vi "UHR-Fleezers Control (host) - 12.0_test_fpga_connection.vi"() -> ()   [LabVIEW 2014] (continued)
              n285 = Add(x=w488, y="Osc. center (V)") -> (x+y=w486:dbl)
              n286 = Divide(x=w486, y=10.0) -> (x/y=w484:dbl)
              n287 = Multiply(x=w484, y=32767.0) -> (x*y=w479:dbl)
              n288 = Select(t=w479, s="Scan axis", f=w499) -> (s? t:f=w497:dbl)
              n289 = Select(t=w498, s="Scan axis", f=w479) -> (s? t:f=w496:dbl)
              n290 = local read "MCL Mode"() -> (w478:u16)
              n291 = Not Equal?(x=w478, y=u16 1) -> (x != y?=w475:bool)
              n292 = local read "Stop All"() -> (w476:bool)
              n293 = xnode "Read/Write Control"("FPGA VI Reference In"=w512, "AO1"=w497, "AO2"=w496) -> ()  [unwired: 1 in, 2 out]
              n294 = Compound Arithmetic op=OR(w476, w475) -> (w474:bool)
              n295 = node-c288() -> ()  [unwired: 2 out]
            }
            n296 = node-c288(w472) -> ()  [unwired: 1 out]
          }
          frame 2 {
            n297 = case shown="True" "Start Scan" {
              tunnel: w518 -> [_ w530]
              frame False {
              }
              frame True {
                n298 = Subtract(x="End (V)", y="Begin (V)") -> (x-y=w526:dbl)
                n299 = Decrement(x="N Points") -> (x-1=w525:dbl)
                n300 = Divide(x=w526, y=w525) -> (x/y=w523:dbl)
                n301 = for {
                  N: "N Points" -> [_]
                  tunnel: "Begin (V)" -> [w543]
                  tunnel: w530 -> [w535]
                  tunnel: [w534] -> w529 mode=indexing
                  tunnel: w523 -> [w533]
                  tunnel: [w531] -> w522 mode=indexing
                  i -> [w542]
                  n302 = Multiply(x=w533, y=w542) -> (x*y=w541:dbl)
                  n303 = Add(x=w543, y=w541) -> (x+y=w538:dbl)
                  n304 = local read "Scan axis"() -> (w532:bool)
                  n305 = local read "AO1"() -> (w540:dbl)
                  n306 = local read "AO2"() -> (w539:dbl)
                  n307 = Select(t=w538, s=w532, f=w540) -> (s? t:f=w537:dbl)
                  n308 = Select(t=w539, s=w532, f=w538) -> (s? t:f=w536:dbl)
                  n309 = flat-sequence {
                    tunnel: w537 -> [w547]
                    tunnel: w536 -> [w546]
                    tunnel: w535 -> [w544]
                    tunnel: [w557] -> w534
                    tunnel: [w556] -> w531
                    frame #0 {
                      w550 = 10.0 ("y")
                      w545 = 32767.0 ("y")
                      n310 = Multiply(x=w547, y=w545) -> (x*y=w553:dbl)
                      n311 = Multiply(x=w546, y=w545) -> (x*y=w551:dbl)
                      n312 = Divide(x=w553, y=w550) -> (x/y=w554:dbl)
                      n313 = Divide(x=w551, y=w550) -> (x/y=w552:dbl)
                      n314 = To Word Integer(number=w554) -> (16bit integer=w548:i16)
                      n315 = To Word Integer(number=w552) -> (16bit integer=w549:i16)
                      n316 = xnode "Read/Write Control"("FPGA VI Reference In"=w544, "AO1"=w548, "AO2"=w549) -> ()  [unwired: 1 in, 2 out]
                    }
                    frame #1 {
                      n317 = Wait (ms)(milliseconds to wait="DAQ Delay (ms)") -> ()  [unwired: 1 out]
                    }
                    frame #2 {
                      n318 = local read "Slow mean"() -> (w557:dbl)
                      n319 = local read "Sigma"() -> (w556:dbl)
                    }
                  }
                }
                n320 = Bundle("Begin (V)"="Begin (V)", w523, w529) -> (→"MCL Scan":cluster{"Begin (V)":dbl, dbl, dbl[]})  [unwired: 1 out]
                n321 = Bundle("Begin (V)"="Begin (V)", w523, w522) -> (→"MCL Scan 2":cluster{"Begin (V)":dbl, dbl, dbl[]})  [unwired: 1 out]
              }
            }
          }
        }
        n322 = local read "Stop All"() -> (w467:bool)
        n323 = node-c288() -> ()  [unwired: 2 out]
      }
      n324 = node-c288(w464) -> ()  [unwired: 1 out]
    }
    frame Enabled {
    }
  }
  n325 = node-c288(3 ("Processor")) -> (w135:T26)  [unwired: 3 out]
  n326 = timed-loop "Oscillate Trap/AOM (fishing, debugging)" {
    tunnel: w51 -> [w561]
    tunnel: [w560] -> w140
    timing: w135 -> [_]
    timing-out: [_] -> w134
    stop <- w560 stop-if-true
    n327 = node-c288() -> ()  [unwired: 2 out]
    n328 = event shown="[0] \"Oscillate Set 1\", \"Fish\": Value Change" {
      selector: _ -> [_ _ _]
      dyn-events: _ -> [_ _ _]
      timeout: _ -> [_ _ _]
      tunnel: w561 -> [w568 _ _]
      tunnel: [FALSE ("Stop All") _ w1253] -> w560
      event "Oscillate Set 1", "Fish": Value Change {
        n329 = event-data() -> ()  [unwired: 6 out]
        n330 = local read "Oscillate Set 1"() -> (w567:bool)
        n331 = Or(x=w567, y="Fish") -> (x .or. y?=w565:bool)
        n332 = case shown="True" w565 {
          tunnel: w568 -> [_ w571]
          tunnel: "Fish" -> [_ w569]
          frame False {
          }
          frame True {
            n333 = case shown="True" w569 {
              selector: w569 -> [w574 w575]
              tunnel: [w574 w575] -> w570
              frame False {
              }
              frame True {
                w576 = FALSE ("Tether")
                n334 = local write "Scan axis 2"(TRUE) -> ()
                n335 = local write "Tether"(w576) -> ()
                n336 = local write "Hysteresis"(w576) -> ()
                n337 = local write "Multiple tether"(w576) -> ()
                n338 = local write "Bad fit"(w576) -> ()
                n339 = local write "Good tether"(w576) -> ()
                n340 = property on="Trap D (MHz)" class="DigNum (strict)"("Val(Sgnl)"="Furthest D (MHz)") -> ()  [unwired: 2 in, 2 out]
                n341 = local read "Flow ON\nduring cal?"() -> (w577:bool)
                n342 = Or(x="Flow ON during \nfishing?", y=w577) -> (x .or. y?=w578:bool)
                n343 = Wait (ms)(milliseconds to wait=u32 500) -> ()  [unwired: 1 out]
                n344 = property on="Sample Channel\nFlow" class="Bool (strict)"("Val(Sgnl)"=w578) -> ()  [unwired: 2 in, 2 out]
              }
            }
            n345 = node-c288() -> (w573:T26)  [unwired: 4 out]
            n346 = timed-loop "Oscillate AOD" {
              timing: w573 -> [_]
              timing-out: [_] -> w572
              tunnel: w571 -> [w590]
              tunnel: w570 -> [w584]
              i -> [w592]
              stop <- w583 stop-if-true
              n347 = node-c288() -> (w591:i64)  [unwired: 1 out]
              n348 = flat-sequence {
                tunnel: w592 -> [w619]
                tunnel: w591 -> [w618]
                tunnel: w590 -> [w597]
                tunnel: w584 -> [w600]
                tunnel: [w600] -> w589
                tunnel: [w599] -> w588
                tunnel: [w596] -> w587
                tunnel: [w593] -> w585
                tunnel: w589 -> [w662]
                tunnel: w588 -> [w660]
                tunnel: w587 -> [w659]
                tunnel: [w658] -> w586
                tunnel: w585 -> [w657]
                tunnel: [w818] -> w583
                tunnel: w586 -> [w817]
                frame #0 {
                  n349 = Divide(x=w618, y=i64 1000) -> (x/y=w613:dbl)
                  n350 = Multiply(x=w613, y=w619) -> (x*y=w615:dbl)
                  n351 = local read "BD 1 Frequency 2 (MHz)"() -> (w598:dbl)
                  n352 = Multiply(x="Osc. freq. (Hz)", y=6.283185307179586) -> (x*y=w616:dbl)
                  n353 = Multiply(x=w616, y=w615) -> (x*y=w595:dbl)
                  n354 = local read "BD 1 Frequency 1 (MHz)"() -> (w603:dbl)
                  n355 = local read "BD 2 Frequency 1 (MHz)"() -> (w602:dbl)
                  n356 = case shown="True" w600 {
                    tunnel: w595 -> [w625 w630]
                    tunnel: w603 -> [_ w641]
                    tunnel: w598 -> [_ w642]
                    tunnel: [w622 w636] -> w601
                    tunnel: [FALSE w633] -> w596
                    tunnel: [0.0 w626] -> w593
                    frame False {
                      n357 = Sine(x=w625) -> (sin(x)=w623:dbl)
                      n358 = Multiply(x=w623, y="Osc. amp. (MHz)") -> (x*y=w622:dbl)
                    }
                    frame True {
                      n359 = Cosine(x=w630) -> (cos(x)=w645:dbl)
                      n360 = Subtract(x=w642, y=w641) -> (x-y=w640:dbl)
                      n361 = Decrement(x=w645) -> (x-1=w644:dbl)
                      n362 = Subtract(x=w640, y="Closest D (MHz)") -> (x-y=w637:dbl)
                      n363 = Divide(x=w644, y=-2.0) -> (x/y=w638:dbl)
                      n364 = Multiply(x=w638, y=w637) -> (x*y=w636:dbl)
                      n365 = local read "Vec Mean of T1 T2"() -> (w632:dbl[])
                      n366 = Greater?(x=w632, y="Stop F (pN)") -> (0:w634:bool[])
                      n367 = Or Array Elements(Boolean array=w634) -> (logical OR=w633:bool)
                      n368 = Divide(x=w630, y=6.283185307179586) -> (x/y=w629:dbl)
                      n369 = Round Toward +Infinity(x=w629) -> (ceil(x): smallest int >= x=w626:dbl)
                      "Attempts" <- w626
                      n370 = Greater?(x=w626, y="Attempt Limit") -> (0:w628:bool)
                      n371 = case shown="True" w628 {
                        frame False {
                        }
                        frame True {
                          n372 = local write "Fish"(FALSE ("Fish for Tether")) -> ()
                          n373 = local read "Messages"() -> (w647:string)
                          n374 = flat-sequence {
                            frame #0 {
                              n375 = call <vilib>:"Beep.vi"("use system alert? (T)"=FALSE, "duration (msec)"=u32 200, "frequency (Hz)"=u32 500) -> ()  [unwired: 9 out]
                            }
                            frame #1 {
                              n376 = Wait (ms)(milliseconds to wait=u32 100) -> ()  [unwired: 1 out]
                            }
                            frame #2 {
                              n377 = call <vilib>:"Beep.vi"("use system alert? (T)"=FALSE, "duration (msec)"=u32 200, "frequency (Hz)"=u32 500) -> ()  [unwired: 9 in]
                            }
                          }
                          n378 = call "Update messages.vi"("Message to add"="Tether fishing timeout." ("Messages"), "Old message string"=w647) -> ("New message string"=→"Messages":string)
                        }
                      }
                    }
                  }
                  n379 = Select(t=w603, s="Scan axis 2", f=w602) -> (s? t:f=w606:dbl)
                  n380 = Add(x=w601, y=w606) -> (x+y=w599:dbl)
                  n381 = Select(t=w599, s="Scan axis 2", f=w603) -> (s? t:f=w609:dbl)
                  n382 = Select(t=w602, s="Scan axis 2", f=w599) -> (s? t:f=w608:dbl)
                  n383 = local read "Y RF Frequency Limits (MHz)"() -> (w604:T17)
                  n384 = local read "X RF Frequency Limits (MHz)"() -> (w605:T17)
                  n385 = local read "BD 2 Frequency 2 (MHz)"() -> (w611:dbl)
                  n386 = local read "BD 2 Frequency 3 (MHz)"() -> (w610:dbl)
                  n387 = local read "BD 1 Frequency 3 (MHz)"() -> (w612:dbl)
                  n388 = call "set RF board frequency - interlace.vi"("Board 2 Frequency Limits"=w604, "Board 1 Frequency Limits"=w605, "FPGA VI Reference In"=w597, "Board 2 Frequency 3 (MHz)"=w610, "Board 1 Frequency 3 (MHz)"=w612, "Board 2 Frequency 2 (MHz)"=w611, "Board 2 Frequency 1 (MHz)"=w608, "Board 1 Frequency 2 (MHz)"=w598, "Board 1 Frequency 1  (MHz)"=w609) -> ()  [unwired: 1 in, 2 out]
                }
                frame #1 {
                  n389 = And(x=w662, y=w659) -> (x .and. y?=w661:bool)
                  n390 = case "Only if were fishing and now formed tether" shown="True" w661 {
                    tunnel: w660 -> [w664 w679]
                    tunnel: [w663 w678] -> w658
                    tunnel: w657 -> [_ w674]
                    frame False {
                      n391 = local read "Fish"() -> (w663:bool)
                      n392 = case shown="False" w663 {
                        tunnel: w664 -> [w665 _]
                        frame False {
                          n393 = property on="BD 1 Frequency 1 (MHz)" class="DigNum (strict)"("Val(Sgnl)"=w665) -> ()  [unwired: 2 in, 2 out]
                        }
                        frame True {
                        }
                      }
                    }
                    frame True {
                      w678 = FALSE ("Fish for Tether")
                      n394 = call <vilib>:"Beep.vi"() -> ()  [unwired: 3 in, 9 out]
                      n395 = Number To Decimal String(number=w674, width (-)=i16 1) -> (decimal integer string=w672:string)
                      n396 = Concatenate Strings("Formed tether in ", w672, " attempt(s)." ("string")) -> (w669:string)
                      n397 = local read "Messages"() -> (w676:string)
                      n398 = local write "Fish"(w678) -> ()
                      n399 = call "Update messages.vi"("Message to add"=w669, "Old message string"=w676) -> ("New message string"=w675:string)
                      n400 = local write "Messages"(w675) -> ()
                      n401 = Get Date/Time In Seconds() -> (seconds since 1Jan1904=→"Time tether formed":timestamp)
                      n402 = local read "Flow ON\nduring cal?"() -> (w666:bool)
                      n403 = property on="Sample Channel\nFlow" class="Bool (strict)"("Val(Sgnl)"=w666) -> (error out=w667:errorcluster)  [unwired: 2 in, 1 out]
                      n404 = case shown="\"2\", \"3\", \"4\", \"5\", \"6\"" "Then..." {
                        selector: "Then..." -> [_ w682 _ _]
                        tunnel: w679 -> [w681 _ _ _]
                        tunnel: w667 -> [_ _ _ _]
                        frame "1", Default {
                          n405 = property on="BD 1 Frequency 1 (MHz)" class="DigNum (strict)"("Val(Sgnl)"=w681) -> ()  [unwired: 2 in, 2 out]
                        }
                        frame "2", "3", "4", "5", "6" {
                          n406 = flat-sequence {
                            tunnel: w682 -> [w688]
                            frame #0 {
                              n407 = local read "Flow ON\nduring cal?"() -> (w683:bool)
                              n408 = property on="Sample Channel\nFlow" class="Bool (strict)"("Val(Sgnl)"=w683) -> ()  [unwired: 2 in, 2 out]
                              n409 = property on="Trap D (MHz)" class="DigNum (strict)"("Val(Sgnl)"="Move to D 1 (MHz)") -> ()  [unwired: 2 in, 2 out]
                            }
                            frame #1 {
                              n410 = local read "Wait Before Save (s)"() -> (w685:u32)
                              n411 = Multiply(x=u32 1000 ("milliseconds to wait"), y=w685) -> (x*y=w687:u32)
                              n412 = Wait (ms)(milliseconds to wait=w687) -> ()  [unwired: 1 out]
                            }
                            frame #2 {
                              n413 = case shown="\"5\", \"6\"" w688 {
                                selector: w688 -> [w691 w701 _]
                                frame "3", "4" {
                                n414 = flat-sequence {
                                tunnel: w691 -> [w692]
                                tunnel: [w692] -> w689
                                tunnel: [w694] -> w690
                                tunnel: w689 -> [w694]
                                tunnel: w690 -> [w698]
                                frame #0 {
                                n415 = property on="Green ON/Interlacing" class="Bool (strict)"("Val(Sgnl)"=TRUE ("Value (Signaling)")) -> ()  [unwired: 2 in, 2 out]
                                }
                                frame #1 {
                                n416 = Multiply(x="Wait Before Save (s)", y=u32 1000 ("x")) -> (x*y=w696:u32)
                                n417 = Wait (ms)(milliseconds to wait=w696) -> ()  [unwired: 1 out]
                                }
                                frame #2 {
                                n418 = property on="Start Saving" class="Bool (strict)"("Value"=TRUE ("Start Saving")) -> ()  [unwired: 2 in, 2 out]
                                n419 = case shown="\"4\"" w698 {
                                frame Default {
                                }
                                frame "4" {
                                n420 = property on="Fl. Triggered..." class="Bool (strict)"("Val(Sgnl)"=TRUE ("Value (Signaling)")) -> ()  [unwired: 2 in, 2 out]
                                }
                                }
                                }
                                }
                                }
                                frame "5", "6" {
                                n421 = stacked-sequence {
                                tunnel: w701 -> [_ _ _ _ _ _ w713]
                                frame #0 {
                                n422 = Replace Array Subset(array=u32[] [0] ("Index Values"), new element="Raster Set\nUpon Tether", index=0) -> (w702:u32[])
                                n423 = property on="Saved AOD Raster Scan Parameter Sets" class="Arr (strict)"("Index Values"=w702) -> ()  [unwired: 2 in, 2 out]
                                }
                                frame #1 {
                                n424 = Wait (ms)(milliseconds to wait=u32 500) -> ()  [unwired: 1 out]
                                }
                                frame #2 {
                                n425 = property on="Load parameters" class="Bool (strict)"("Val(Sgnl)"=TRUE ("Value (Signaling)")) -> ()  [unwired: 2 in, 2 out]
                                n426 = case shown="True" "Green ON during\nraster?" {
                                frame False {
                                }
                                frame True {
                                n427 = property on="Green ON/Interlacing" class="Bool (strict)"("Val(Sgnl)"=TRUE ("Value (Signaling)")) -> ()  [unwired: 2 in, 2 out]
                                }
                                }
                                }
                                frame #3 {
                                n428 = Wait (ms)(milliseconds to wait=u32 500) -> ()  [unwired: 1 out]
                                }
                                frame #4 {
                                n429 = property on="Trap Raster Scan" class="Bool (strict)"("Val(Sgnl)"=TRUE ("Value (Signaling)")) -> ()  [unwired: 2 in, 2 out]
                                }
                                frame #5 {
                                n430 = Wait (ms)(milliseconds to wait=u32 2000) -> ()  [unwired: 1 out]
                                }
                                frame #6 {
                                n431 = flat-sequence {
                                tunnel: w713 -> [w720]
                                frame #0 {
                                n432 = while {
                                stop <- w716 stop-if-true
                                n433 = local read "Raster Scanning..."() -> (w715:bool)
                                n434 = local read "Saving..."() -> (w718:bool)
                                n435 = Wait (ms)(milliseconds to wait=u32 100) -> ()  [unwired: 1 out]
                                n436 = Not(x=w718) -> (.not. x?=w717:bool)
                                n437 = Not(x=w715) -> (.not. x?=w714:bool)
                                n438 = And(x=w717, y=w714) -> (x .and. y?=w716:bool)
                                }
                                }
                                frame #1 {
                                n439 = local read "Tether"() -> (w721:bool)
                                n440 = case shown="True" w721 {
                                tunnel: w720 -> [_ w723]
                                frame False {
                                n441 = property on="Fish" class="Bool (strict)"("Val(Sgnl)"="Fish again after \nraster break?") -> ()  [unwired: 2 in, 2 out]
                                }
                                frame True {
                                n442 = stacked-sequence {
                                tunnel: w723 -> [_ w727 _ _ _ _ _ _]
                                frame #0 {
                                n443 = property on="Trap D (MHz)" class="DigNum (strict)"("Val(Sgnl)"="Move to D 2 (MHz)") -> ()  [unwired: 2 in, 2 out]
                                n444 = case shown="True" "Flow ON after\ntether testing?" {
                                frame False {
                                }
                                frame True {
                                n445 = property on="Sample Channel\nFlow" class="Bool (strict)"("Val(Sgnl)"=TRUE ("Value (Signaling)")) -> ()  [unwired: 2 in, 2 out]
                                }
                                }
                                }
                                frame #1 {
                                n446 = flat-sequence {
                                tunnel: w727 -> [w728]
                                frame #0 {
                                n447 = case shown="\"6\"" w728 {
                                frame Default {
                                }
                                frame "6" {
                                n448 = flat-sequence {
                                frame #0 {
                                n449 = Wait (ms)(milliseconds to wait=u32 500) -> ()  [unwired: 1 out]
                                }
                                frame #1 {
                                n450 = property on="Green ON/Interlacing" class="Bool (strict)"("Val(Sgnl)"=TRUE ("Green Laser ON/Interlacing")) -> ()  [unwired: 2 in, 2 out]
                                }
                                }
                                }
                                }
                                }
                                frame #1 {
                                n451 = case shown="True" "Save at end (5, 6)" {
                                selector: "Save at end (5, 6)" -> [_ w732]
                                frame False {
                                }
                                frame True {
                                n452 = flat-sequence {
                                tunnel: w732 -> [w734]
                                frame #0 {
                                n453 = Wait (ms)(milliseconds to wait=u32 500) -> ()  [unwired: 1 out]
                                }
                                frame #1 {
                                n454 = local write "Start Saving"(w734) -> ()
                                }
                                }
                                }
                                }
                                }
                                }
                                }
                                frame #2 {
                                n455 = local read "Bead Sep. Int. Time (s)"() -> (w737:dbl)
                                n456 = Multiply(x=w737, y=1000.0) -> (x*y=w736:dbl)
                                n457 = Wait (ms)(milliseconds to wait=w736) -> ()  [unwired: 1 out]
                                }
                                frame #3 {
                                n458 = property on="Remove Offset" class="Bool (strict)"("Val(Sgnl)"=TRUE ("Value (Signaling)")) -> ()  [unwired: 2 in, 2 out]
                                }
                                frame #4 {
                                n459 = property on="Read FX file" class="Bool (strict)"("Val(Sgnl)"=TRUE ("Value (Signaling)")) -> ()  [unwired: 2 in, 2 out]
                                }
                                frame #5 {
                                n460 = Wait (ms)(milliseconds to wait=u32 300) -> ()  [unwired: 1 out]
                                }
                                frame #6 {
                                n461 = local read "Bad fit error"() -> (w746:dbl)
                                n462 = local read "Fit offset"() -> (w749:dbl)
                                n463 = Greater Or Equal?(x=w746, y="Bad fit thresh") -> (x >= y?=→"Bad fit":bool)
                                n464 = Greater Or Equal?(x=w749, y="Fit offset thresh") -> (x >= y?=→"Multiple tether":bool)
                                n465 = local read "Hyst. error"() -> (w743:dbl)
                                n466 = Greater Or Equal?(x=w743, y="Hysteresis thresh") -> (x >= y?=→"Hysteresis":bool)
                                }
                                frame #7 {
                                w754 = 0
                                n467 = local read "Bad fit error"() -> (w756:dbl)
                                n468 = local read "Hyst. error"() -> (w755:dbl)
                                n469 = local read "Fit offset"() -> (w757:dbl)
                                n470 = local read "Multiple tether"() -> (w763:bool)
                                n471 = local read "Hysteresis"() -> (w761:bool)
                                n472 = local read "Bad fit"() -> (w762:bool)
                                n473 = Not(x=w761) -> (.not. x?=w753:bool)
                                n474 = Not(x=w762) -> (.not. x?=w759:bool)
                                n475 = Greater?(x=w757, y=w754) -> (0:w752:bool)
                                n476 = Greater?(x=w756, y=w754) -> (0:w751:bool)
                                n477 = Greater?(x=w755, y=w754) -> (0:w750:bool)
                                n478 = Not(x=w763) -> (.not. x?=w760:bool)
                                n479 = Compound Arithmetic op=AND(w760, w759, w753, w752, w751, w750) -> (w758:bool)
                                "Good tether" <- w758
                                n480 = case shown="True" w758 {
                                frame False {
                                }
                                frame True {
                                n481 = call <vilib>:"Beep.vi"("use system alert? (T)"=FALSE, "duration (msec)"=u32 200, "frequency (Hz)"=u32 2000) -> ()  [unwired: 9 in]
                                }
                                }
                                }
                                }
                                }
                                }
                                }
                                }
                                }
                                }
                                }
                                frame "2", Default {
                                }
                              }
                            }
                            frame #3 {
                              n482 = local read "Multiple tether"() -> (w769:bool)
                              n483 = And(x="Break multiple", y=w769) -> (x .and. y?=w767:bool)
                              n484 = case shown="True" w767 {
                                frame False {
                                }
                                frame True {
                                n485 = stacked-sequence {
                                frame #0 {
                                n486 = property on="Trap D (MHz)" class="DigNum (strict)"("Val(Sgnl)"="Trap D to \nbreak (MHz)") -> ()  [unwired: 2 in, 2 out]
                                }
                                frame #1 {
                                n487 = case shown="True" "Fish after\nmultiple break" {
                                frame False {
                                }
                                frame True {
                                n488 = while {
                                stop <- w774 stop-if-true
                                n489 = local read "Multiple tether"() -> (w776:bool)
                                n490 = local read "Fish"() -> (w773:bool)
                                n491 = local read "Stop All"() -> (w772:bool)
                                n492 = Wait (ms)(milliseconds to wait=u32 100) -> ()  [unwired: 1 out]
                                n493 = Not(x=w776) -> (.not. x?=w775:bool)
                                n494 = Compound Arithmetic op=OR(w772, w775, w773) -> (w774:bool)
                                }
                                }
                                }
                                }
                                frame #2 {
                                n495 = local read "Fish after\nmultiple break"() -> (w781:bool)
                                n496 = local read "Stage Moving"() -> (w780:bool)
                                n497 = Not(x=w780) -> (.not. x?=w778:bool)
                                n498 = And(x=w781, y=w778) -> (x .and. y?=w779:bool)
                                n499 = property on="Fish" class="Bool (strict)"("Val(Sgnl)"=w779) -> ()  [unwired: 2 in, 2 out]
                                }
                                }
                                }
                              }
                            }
                            frame #4 {
                              n500 = local read "Bad fit"() -> (w783:bool)
                              n501 = And(x="Break bad fit", y=w783) -> (x .and. y?=w782:bool)
                              n502 = case shown="True" w782 {
                                frame False {
                                }
                                frame True {
                                n503 = stacked-sequence {
                                frame #0 {
                                n504 = local read "Trap D to \nbreak (MHz)"() -> (w785:dbl)
                                n505 = property on="Trap D (MHz)" class="DigNum (strict)"("Val(Sgnl)"=w785) -> ()  [unwired: 2 in, 2 out]
                                }
                                frame #1 {
                                n506 = case shown="True" "Fish after\nbad fit break?" {
                                frame False {
                                }
                                frame True {
                                n507 = while {
                                stop <- w789 stop-if-true
                                n508 = local read "Stop All"() -> (w787:bool)
                                n509 = local read "Bad fit"() -> (w788:bool)
                                n510 = local read "Fish"() -> (w790:bool)
                                n511 = Not(x=w788) -> (.not. x?=w791:bool)
                                n512 = Wait (ms)(milliseconds to wait=u32 100) -> ()  [unwired: 1 out]
                                n513 = Compound Arithmetic op=OR(w787, w791, w790) -> (w789:bool)
                                }
                                }
                                }
                                }
                                frame #2 {
                                n514 = local read "Fish after\nbad fit break?"() -> (w793:bool)
                                n515 = local read "Stage Moving"() -> (w796:bool)
                                n516 = Not(x=w796) -> (.not. x?=w795:bool)
                                n517 = And(x=w793, y=w795) -> (x .and. y?=w794:bool)
                                n518 = property on="Fish" class="Bool (strict)"("Val(Sgnl)"=w794) -> ()  [unwired: 2 in, 2 out]
                                }
                                }
                                }
                              }
                            }
                            frame #5 {
                              n519 = local read "Hysteresis"() -> (w798:bool)
                              n520 = And(x="Break hyst", y=w798) -> (x .and. y?=w797:bool)
                              n521 = case shown="True" w797 {
                                frame False {
                                }
                                frame True {
                                n522 = stacked-sequence {
                                frame #0 {
                                n523 = local read "Trap D to \nbreak (MHz)"() -> (w800:dbl)
                                n524 = property on="Trap D (MHz)" class="DigNum (strict)"("Val(Sgnl)"=w800) -> ()  [unwired: 2 in, 2 out]
                                }
                                frame #1 {
                                n525 = case shown="True" "Fish ater hyst?" {
                                frame False {
                                }
                                frame True {
                                n526 = while {
                                stop <- w806 stop-if-true
                                n527 = local read "Hysteresis"() -> (w805:bool)
                                n528 = local read "Stop All"() -> (w802:bool)
                                n529 = local read "Fish"() -> (w803:bool)
                                n530 = Wait (ms)(milliseconds to wait=u32 100) -> ()  [unwired: 1 out]
                                n531 = Not(x=w805) -> (.not. x?=w804:bool)
                                n532 = Compound Arithmetic op=OR(w802, w804, w803) -> (w806:bool)
                                }
                                }
                                }
                                }
                                frame #2 {
                                n533 = local read "Fish ater hyst?"() -> (w811:bool)
                                n534 = local read "Stage Moving"() -> (w810:bool)
                                n535 = Not(x=w810) -> (.not. x?=w809:bool)
                                n536 = And(x=w811, y=w809) -> (x .and. y?=w808:bool)
                                n537 = property on="Fish" class="Bool (strict)"("Val(Sgnl)"=w808) -> ()  [unwired: 2 in, 2 out]
                                }
                                }
                                }
                              }
                            }
                            frame #6 {
                              n538 = local read "Good tether"() -> (w812:bool)
                              n539 = case shown="True" w812 {
                                frame False {
                                }
                                frame True {
                                n540 = case shown="\"1\"" "If good, then:" {
                                frame "0", Default {
                                }
                                frame "1" {
                                n541 = property on="Force FB Script" class="Bool (strict)"("Val(Sgnl)"=TRUE ("Value (Signaling)")) -> ()  [unwired: 2 in, 2 out]
                                }
                                }
                                }
                              }
                            }
                          }
                        }
                        frame "7" {
                          n542 = property on="Force FB Script" class="Bool (strict)"("Val(Sgnl)"=TRUE ("Value (Signaling)")) -> ()  [unwired: 2 in, 2 out]
                        }
                        frame "8" {
                          n543 = property on="Fixed Traps Script" class="Bool (strict)"("Val(Sgnl)"=TRUE ("Value (Signaling)")) -> ()  [unwired: 2 in, 2 out]
                        }
                      }
                      "Tether" <- "Tether Alarm?"
                    }
                  }
                }
                frame #2 {
                  n544 = local read "Oscillate Set 1"() -> (w822:bool)
                  n545 = local read "Stop All"() -> (w820:bool)
                  n546 = Or(x=w822, y=w817) -> (x .or. y?=w819:bool)
                  n547 = Not(x=w819) -> (.not. x?=w821:bool)
                  n548 = Compound Arithmetic op=OR(w820, w821) -> (w818:bool)
                }
              }
              n549 = node-c288() -> ()  [unwired: 2 out]
            }
            n550 = node-c288(w572) -> ()  [unwired: 1 out]
          }
        }
      }
      event "Fl. Triggered...": Value Change {
        n551 = event-data() -> ()  [unwired: 7 out]
        n552 = case shown="True" "Fl. Triggered..." {
          frame False {
          }
          frame True {
            n553 = node-c288() -> (w833:T26)  [unwired: 4 out]
            n554 = timed-loop {
              timing: w833 -> [_]
              timing-out: [_] -> w832
              tunnel: "Action" -> [w841]
              shift-right: [w838] -> _
              shift-left: u8 255 -> [w840]
              shift-right: [w835] -> _
              shift-left: 255 -> [w837]
              stop <- w834 stop-if-true
              # "Reset confocal spot"
              n555 = node-c288() -> ()  [unwired: 2 out]
              n556 = flat-sequence {
                tunnel: w841 -> [w861]
                tunnel: w840 -> [w860]
                tunnel: [w859] -> w839
                tunnel: w837 -> [w846]
                tunnel: [w845] -> w836
                tunnel: [w1245] -> w834
                tunnel: w839 -> [w1244]
                tunnel: [w1244] -> w838
                tunnel: [w1243] -> w835
                tunnel: w836 -> [w1243]
                frame #0 {
                  n557 = local read "Delta Fl. 2"() -> (w858:dbl)
                  n558 = local read "Delta Fl. 1"() -> (w853:dbl)
                  n559 = Multiply(x="Fl. D Thresh. (kHz)", y=1000.0) -> (x*y=w848:dbl)
                  n560 = Select(t=w853, s="APD to Watch", f=w858) -> (s? t:f=w849:dbl)
                  n561 = Greater?(x=w849, y=w848) -> (0:w854:bool)
                  n562 = Or(x="Force Yank", y=w854) -> (x .or. y?=w852:bool)
                  n563 = And(x=w852, y="Yank when?") -> (x .and. y?=w850:bool)
                  n564 = case shown="False" w850 {
                    tunnel: w861 -> [w864 w1067]
                    tunnel: w860 -> [w866 w1063]
                    tunnel: [w866 w1061] -> w859
                    tunnel: w849 -> [w872 _]
                    tunnel: w848 -> [w871 _]
                    tunnel: "Force Yank" -> [w869 _]
                    tunnel: w846 -> [w868 w1060]
                    tunnel: [w867 w1060] -> w845
                    frame False {
                      n565 = Negate(x=w871) -> (-x=w863:dbl)
                      n566 = local write "Fl. High"(TRUE ("Fl. High")) -> ()
                      n567 = Less?(x=w872, y=w863) -> (x < y?=w870:bool)
                      n568 = Or(x=w869, y=w870) -> (x .or. y?=w865:bool)
                      n569 = case shown="True" w865 {
                        tunnel: w868 -> [w873 w883]
                        tunnel: [w873 w882] -> w867
                        tunnel: w864 -> [_ w881]
                        frame False {
                        }
                        frame True {
                          n570 = flat-sequence {
                            tunnel: w883 -> [w889]
                            tunnel: w881 -> [w886]
                            tunnel: [w888] -> w880
                            tunnel: [w887] -> w879
                            tunnel: [w886] -> w878
                            tunnel: w877 -> [w885]
                            tunnel: [w885] -> w876
                            tunnel: w875 -> [w884]
                            tunnel: [w884] -> w874
                            tunnel: [w961] -> w882
                            tunnel: w880 -> [w961]
                            tunnel: w879 -> [w960]
                            tunnel: w878 -> [w959]
                            tunnel: w876 -> [w958]
                            tunnel: w874 -> [w957]
                            frame #0 {
                              n571 = call <vilib>:"Beep.vi"() -> ()  [unwired: 12 in]
                              n572 = local write "Waiting"(FALSE ("Waiting")) -> ()
                              n573 = Increment(x=w889) -> (x+1=w888:i32)
                              n574 = case shown="\"Yank\"" w886 {
                                tunnel: w888 -> [_ w894 _]
                                frame "Alarm", Default {
                                }
                                frame "Yank" {
                                n575 = flat-sequence {
                                tunnel: w894 -> [w897]
                                tunnel: [w896] -> w893
                                tunnel: [w895] -> w892
                                tunnel: w893 -> [w907]
                                tunnel: w892 -> [w908]
                                frame #0 {
                                n576 = local read "Yank Delay (s)"() -> (w900:dbl)
                                n577 = local read "N Array El"() -> (w895:u8)
                                n578 = Quotient & Remainder(x=w897, y=w895) -> (x-y*floor(x/y)=w896:i32)  [unwired: 1 out]
                                n579 = Multiply(x=w900, y=1000.0) -> (x*y=w898:dbl)
                                n580 = Wait (ms)(milliseconds to wait=w898) -> ()  [unwired: 1 out]
                                }
                                frame #1 {
                                n581 = local read "Yank to which?"() -> (w902:bool)
                                n582 = local read "Random Choice"() -> (w912:bool)
                                n583 = local read "Yank to Trap D (MHz)"() -> (w905:dbl[])
                                n584 = local read "Yank to SP"() -> (w906:dbl[])
                                n585 = Random Number (0-1)() -> (number: 0 to 1=w911:dbl)
                                n586 = Multiply(x=w908, y=w911) -> (x*y=w910:dbl)
                                n587 = Round Toward -Infinity(1:w910) -> (0:w909:dbl)
                                n588 = Select(t=w909, s=w912, f=w907) -> (s? t:f=w903:dbl)
                                n589 = Select(t=w905, s=w902, f=w906) -> (s? t:f=w904:dbl[])
                                n590 = Index Array(array=w904, index=w903) -> (element=w901:dbl)
                                n591 = case shown="False" w902 {
                                tunnel: w901 -> [w913 w941]
                                frame False {
                                n592 = flat-sequence {
                                tunnel: w913 -> [w914]
                                frame #0 {
                                n593 = property on="Trap Pos FB SP" class="DigNum (strict)"("Val(Sgnl)"=w914) -> ()  [unwired: 2 in, 2 out]
                                }
                                frame #1 {
                                n594 = Wait (ms)(milliseconds to wait=u32 700) -> ()  [unwired: 1 out]
                                }
                                frame #2 {
                                n595 = local read "Action (%)"() -> (w919:dbl)
                                n596 = Absolute Value(x=w919) -> (abs(x)=w918:dbl)
                                n597 = Greater?(x=w918, y=70.0) -> (0:w916:bool)
                                n598 = property on="Remove Action Offset" class="Bool (strict)"("Val(Sgnl)"=w916) -> ()  [unwired: 2 in, 2 out]
                                }
                                frame #3 {
                                n599 = for {
                                N: 4 -> [_]
                                n600 = flat-sequence {
                                frame #0 {
                                n601 = Wait (ms)(milliseconds to wait=u32 500) -> ()  [unwired: 1 out]
                                }
                                frame #1 {
                                n602 = local read "Action (%)"() -> (w925:dbl)
                                n603 = Absolute Value(x=w925) -> (abs(x)=w924:dbl)
                                n604 = Greater?(x=w924, y=70.0) -> (0:w922:bool)
                                n605 = property on="Remove Action Offset" class="Bool (strict)"("Val(Sgnl)"=w922) -> ()  [unwired: 2 in, 2 out]
                                }
                                }
                                }
                                }
                                frame #4 {
                                n606 = Wait (ms)(milliseconds to wait=u32 500) -> ()  [unwired: 1 out]
                                }
                                frame #5 {
                                n607 = local read "Mean"() -> (w933:dbl)
                                n608 = Greater?(x=w933, y=11.0) -> (0:w927:bool)
                                n609 = Not(x=w927) -> (.not. x?=w928:bool)
                                n610 = And(x=w928, y="Shift confocal") -> (x .and. y?=w930:bool)
                                n611 = And(x=w927, y="Shift confocal") -> (x .and. y?=w931:bool)
                                n612 = case shown="True" w931 {
                                frame False {
                                }
                                frame True {
                                n613 = local read "Confocal Y 2 (V)"() -> (w937:dbl)
                                n614 = local read "Confocal X 2 (V)"() -> (w936:dbl)
                                n615 = property on="AO1" class="Slide (strict)"("Val(Sgnl)"=w937) -> ()  [unwired: 2 in, 2 out]
                                n616 = property on="AO2" class="Slide (strict)"("Val(Sgnl)"=w936) -> ()  [unwired: 2 in, 2 out]
                                }
                                }
                                n617 = case shown="True" w930 {
                                frame False {
                                }
                                frame True {
                                n618 = local read "Confocal Y 1 (V)"() -> (w935:dbl)
                                n619 = local read "Confocal X 1 (V)"() -> (w934:dbl)
                                n620 = property on="AO1" class="Slide (strict)"("Val(Sgnl)"=w935) -> ()  [unwired: 2 in, 2 out]
                                n621 = property on="AO2" class="Slide (strict)"("Val(Sgnl)"=w934) -> ()  [unwired: 2 in, 2 out]
                                }
                                }
                                }
                                frame #6 {
                                n622 = Wait (ms)(milliseconds to wait=u32 1500) -> ()  [unwired: 1 out]
                                }
                                frame #7 {
                                n623 = property on="Rem fb disp offset" class="Bool (strict)"("Val(Sgnl)"=TRUE ("Value (Signaling)")) -> ()  [unwired: 2 in, 2 out]
                                n624 = property on="Remove Offset" class="Bool (strict)"("Val(Sgnl)"=TRUE ("Value (Signaling)")) -> ()  [unwired: 2 in, 2 out]
                                }
                                }
                                }
                                frame True {
                                n625 = flat-sequence {
                                tunnel: w941 -> [w942]
                                frame #0 {
                                n626 = property on="Trap D (MHz)" class="DigNum (strict)"("Val(Sgnl)"=w942) -> ()  [unwired: 2 in, 2 out]
                                }
                                frame #1 {
                                n627 = Wait (ms)(milliseconds to wait=u32 500) -> ()  [unwired: 1 out]
                                }
                                frame #2 {
                                n628 = local read "Shift confocal"() -> (w948:bool)
                                n629 = local read "Mean"() -> (w950:dbl)
                                n630 = Greater?(x=w950, y=11.0) -> (0:w947:bool)
                                n631 = Not(x=w947) -> (.not. x?=w946:bool)
                                n632 = And(x=w946, y=w948) -> (x .and. y?=w944:bool)
                                n633 = And(x=w947, y=w948) -> (x .and. y?=w945:bool)
                                n634 = case shown="True" w945 {
                                frame False {
                                }
                                frame True {
                                n635 = local read "Confocal Y 2 (V)"() -> (w954:dbl)
                                n636 = local read "Confocal X 2 (V)"() -> (w953:dbl)
                                n637 = property on="AO2" class="Slide (strict)"("Val(Sgnl)"=w953) -> ()  [unwired: 2 in, 2 out]
                                n638 = property on="AO1" class="Slide (strict)"("Val(Sgnl)"=w954) -> ()  [unwired: 2 in, 2 out]
                                }
                                }
                                n639 = case shown="True" w944 {
                                frame False {
                                }
                                frame True {
                                n640 = local read "Confocal X 1 (V)"() -> (w951:dbl)
                                n641 = local read "Confocal Y 1 (V)"() -> (w952:dbl)
                                n642 = property on="AO2" class="Slide (strict)"("Val(Sgnl)"=w951) -> ()  [unwired: 2 in, 2 out]
                                n643 = property on="AO1" class="Slide (strict)"("Val(Sgnl)"=w952) -> ()  [unwired: 2 in, 2 out]
                                }
                                }
                                }
                                }
                                }
                                }
                                }
                                }
                                }
                                frame "Image" {
                                n644 = property on="Confocal\nImage" class="Bool (strict)"("Val(Sgnl)"=TRUE ("Value (Signaling)")) -> ()  [unwired: 2 in, 2 out]
                                }
                              }
                              n645 = local write "Fl. High"(FALSE ("Fl. High")) -> ()
                              n646 = local read "Time (s)"() -> (w887:dbl)
                            }
                            frame #1 {
                              n647 = case shown="True" "Auto F Reset" {
                                tunnel: w960 -> [_ w965]
                                tunnel: w959 -> [_ w964]
                                tunnel: w958 -> [_ w963]
                                tunnel: w957 -> [_ w962]
                                frame False {
                                }
                                frame True {
                                n648 = node-c288() -> (w967:T26)  [unwired: 4 in]
                                n649 = timed-loop {
                                timing: w967 -> [_]
                                timing-out: [_] -> w966
                                tunnel: w965 -> [w972]
                                tunnel: w964 -> [w971]
                                tunnel: w963 -> [w970]
                                tunnel: w962 -> [w969]
                                stop <- w968 stop-if-true
                                n650 = node-c288() -> ()  [unwired: 1 in, 1 out]
                                n651 = local read "APD to Watch"() -> (w982:bool)
                                n652 = local read "Fl. D Thresh. (kHz)"() -> (w981:dbl)
                                n653 = local read "Delta Fl. 1"() -> (w983:dbl)
                                n654 = local read "Delta Fl. 2"() -> (w984:dbl)
                                n655 = local read "Fl. Triggered..."() -> (w975:bool)
                                n656 = local read "Stop All"() -> (w976:bool)
                                n657 = local read "Reset Force"() -> (w974:bool)
                                n658 = Multiply(x=w981, y=1000.0) -> (x*y=w979:dbl)
                                n659 = Not(x=w975) -> (.not. x?=w973:bool)
                                n660 = Select(t=w983, s=w982, f=w984) -> (s? t:f=w978:dbl)
                                n661 = Greater?(x=w978, y=w979) -> (0:w977:bool)
                                n662 = Compound Arithmetic op=OR(w977, w976, w973, w974) -> (w968:bool)
                                n663 = case shown="True" w968 {
                                tunnel: w972 -> [_ w988]
                                tunnel: w971 -> [_ w992]
                                tunnel: w970 -> [_ w991]
                                tunnel: w969 -> [_ w990]
                                frame False {
                                }
                                frame True {
                                n664 = case shown="\"Yank\"" w992 {
                                tunnel: w991 -> [_ w1002]
                                tunnel: w990 -> [_ w1000]
                                frame "Image", Default {
                                }
                                frame "Yank" {
                                n665 = flat-sequence {
                                tunnel: [w1005] -> w1003
                                tunnel: w1002 -> [w1005]
                                tunnel: [w1004] -> w1001
                                tunnel: w1000 -> [w1004]
                                tunnel: w1003 -> [w1011]
                                tunnel: w1001 -> [w1009]
                                frame #0 {
                                n666 = local read "Yank Delay (s)"() -> (w1008:dbl)
                                n667 = Multiply(x=w1008, y=1000.0) -> (x*y=w1006:dbl)
                                n668 = Wait (ms)(milliseconds to wait=w1006) -> ()  [unwired: 1 out]
                                }
                                frame #1 {
                                n669 = local read "Yank to which?"() -> (w1010:bool)
